vi "Kalibrier_Infos_Auswerten.vi"(11 "Sprachliste":string[][](array[string])) -> (0 "ErrorMessage PDF":string, 1 "Kalibrier Info Text":string, 2 "Kalibrier Infos Array":string[](array[string]), 3 "Kalibrier Error occured":bool)   [LabVIEW 2020, in "Linearisierung v2.lvlib" / "SpanEinstellungen.lvlib"]
uses:
  SpanEinstellungen.lvlib
  Aktion FGV GD Errors sammeln.ctl
  Sprachverwaltung/Sprachverwaltung.lvlib
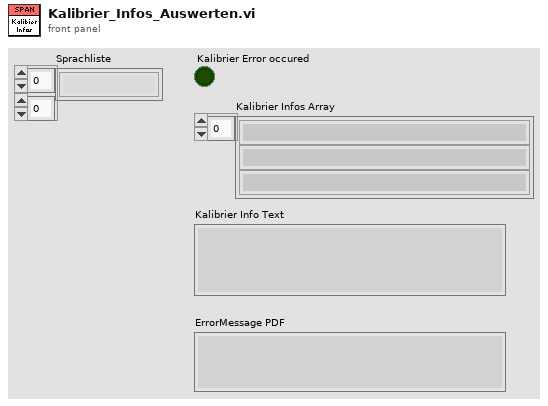
[diagram p1: front panel]
types:
  T1 = typedef "Linearisierung v2.lvlib/SpanEinstellungen.lvlib/Aktion FGV GD Errors sammeln.ctl" = enum16{"lesen", "init", "GD Infos sammeln", "Kalibrierinfos sammeln", "Test Data", "GD Infos selektiv sammeln"}
  T2 = typedef "Linearisierung v2.lvlib/SpanEinstellungen.lvlib/Kalibrier Info Cluster.ctl" = cluster{"Wobei":string, "Calibration succesful":bool, "Value is in the valid range":bool, "Zeitstempel":string}
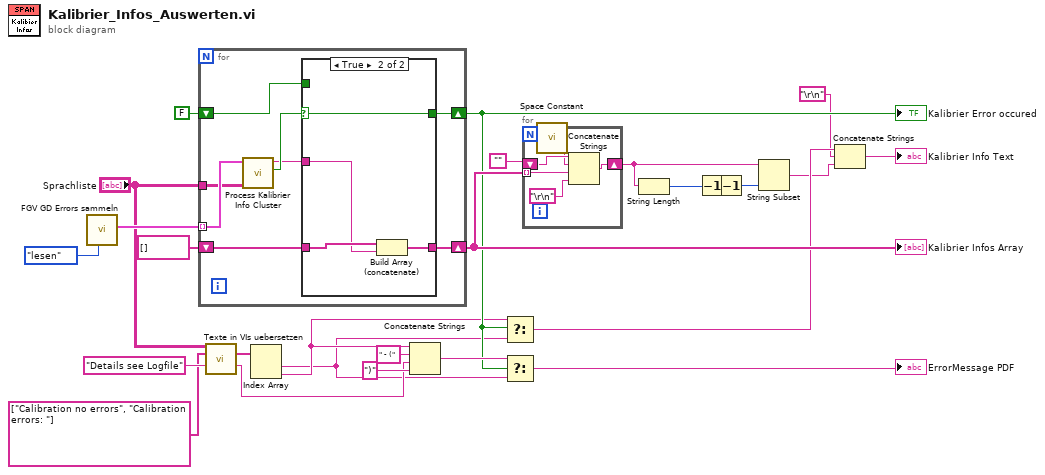
[diagram p0: block diagram]
diagram:
  n1 = call "FGV GD Errors sammeln.vi"("Aktion"=Aktion_FGV_GD_Errors_sammeln."lesen") -> ("Kalibrier Info-Cluster out"=w23:T2[])  [unwired: 8 in, 2 out]
  n2 = for {
    shift-right: [w28] -> w21
    shift-left: string[] [] -> [w34]
    shift-right: [w33] -> w11
    shift-left: FALSE -> [w32]
    tunnel: w23 -> [w31] mode=indexing
    tunnel: "Sprachliste" -> [w27]
    n3 = call "Process Kalibrier Info Cluster.vi"("Sprachliste"=w27, "Kalibrier Info-Cluster in"=w31) -> ("Fehler"=w30:bool, "String"=w29:string)  [unwired: 8 in]
    n4 = case shown="True" w30 {
      selector: w30 -> [_ w38]
      tunnel: [w35 w40] -> w28
      tunnel: w34 -> [w35 w39]
      tunnel: [w36 w38] -> w33
      tunnel: w32 -> [w36 _]
      tunnel: w29 -> [_ w37]
      frame False {
      }
      frame True {
        n5 = Build Array (concatenate)(w39, w37) -> (w40:string[])
      }
    }
  }
  "Kalibrier Infos Array" <- w21
  "Kalibrier Error occured" <- w11
  n6 = call "Texte in VIs uebersetzen.vi"("Sprachliste"="Sprachliste", "String-Array zum Übersetzen"=string[] ["Calibration no errors", "Calibration errors: "] ("t"), "String zum Übersetzen"="Details see Logfile") -> ("String-Array zum Übersetzen"=w13:string[], "String zum Übersetzen"=w12:string)  [unwired: 8 in, 3 out]
  n7 = Index Array(array=w13) -> (element #1=w9:string, element #2=w10:string)  [unwired: 2 in]
  n8 = Concatenate Strings(w10, " - (" ("String"), w12, ")" ("String")) -> (w18:string)
  n9 = Select(t=w10, s=w11, f=w9) -> (s? t:f=w8:string)
  n10 = Select(t=w18, s=w11, f=w9) -> (s? t:f=→"ErrorMessage PDF":string)
  n11 = for {
    tunnel: w21 -> [w45] mode=indexing
    shift-right: [w44] -> w4
    shift-left: "" -> [w43]
    n12 = call <vilib>:"Space Constant.vi"() -> ("String"=w42:string)
    n13 = Concatenate Strings(w43, w42, w45, "\r\n") -> (w44:string)
  }
  n14 = String Length(string=w4) -> (length=w5:i32)
  n15 = Decrement(x=w5) -> (x-1=w1:i32)
  n16 = Decrement(x=w1) -> (x-1=w3:i32)
  n17 = String Subset(string=w4, length (rest)=w3) -> (substring=w2:string)  [unwired: 1 in]
  n18 = Concatenate Strings(w8, "\r\n", w2) -> (→"Kalibrier Info Text":string)
